vi "DHE_InspectName.vi"(10 "name in":string) -> (2 "name out":string)   [LabVIEW 2016]
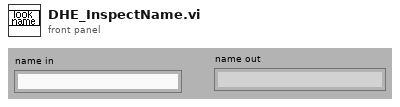
[diagram p1: front panel]
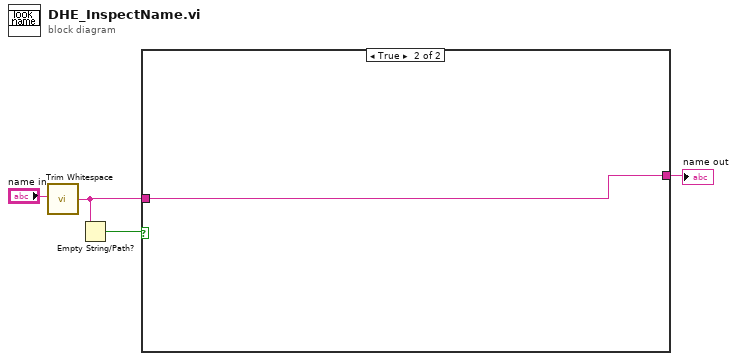
[diagram p0: block diagram]
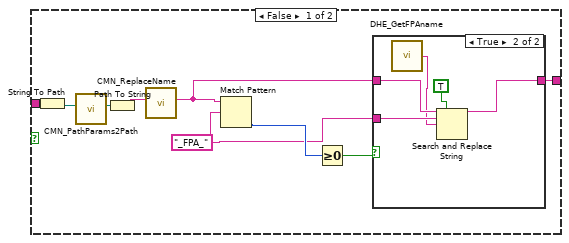
[diagram p2: hidden frame]
diagram:
  n1 = call <vilib>:"Trim Whitespace.vi"("string"="name in") -> ("trimmed string"=w1:string)  [unwired: 1 in]
  n2 = Empty String/Path?(string/path=w1) -> (empty?=w2:bool)
  n3 = case shown="True" w2 {
    tunnel: [w11 w20] -> w4
    tunnel: w1 -> [w5 w20]
    frame False {
      w10 = "_FPA_" ("regular expression")
      n4 = String To Path(string=w5) -> (path=w9:path)
      n5 = call "CMN_PathParams2Path.vi"("Path In"=w9) -> ("Path out"=w8:path)  [unwired: 2 in, 8 out]
      n6 = Path To String(path=w8) -> (string=w7:string)
      n7 = call "CMN_ReplaceName.vi"("name in"=w7) -> ("name out"=w6:string)  [unwired: 1 in, 9 out]
      n8 = Match Pattern(string=w6, regular expression=w10) -> (offset past match=w13:i32)  [unwired: 4 out]
      n9 = Greater Or Equal To 0?(x=w13) -> (x >= 0?=w12:bool)
      n10 = case shown="True" w12 {
        tunnel: w6 -> [w14 w19]
        tunnel: [w14 w16] -> w11
        tunnel: w10 -> [_ w18]
        frame False {
        }
        frame True {
          n11 = call "DHE_GetFPAname.vi"() -> ("DHE_FPAname"=w17:string)  [unwired: 9 out]
          n12 = Search and Replace String(replace all?=TRUE ("replace all? (F)"), input string=w19, search string=w18, replace string=w17) -> (result string=w16:string)  [unwired: 1 in, 6 out]
        }
      }
    }
    frame True {
    }
  }
  "name out" <- w4
